vi "FT_Get_Device_Info.vi"(0 "Handle":u32) -> (1 "FT_Status":u32(ring) items=["FT_OK", "FT_INVALID_HANDLE", "FT_DEVICE_NOT_FOUND", "FT_DEVICE_NOT_OPENED", "FT_IO_ERROR", "FT_INSUFFICIENT_RESOURCES", "FT_INVALID_PARAMETER", "FT_INVALID_BAUD_RATE", "FT_DEVICE_NOT_OPENED_FOR_ERASE", "FT_DEVICE_NOT_OPENED_FOR_WRITE", "FT_FAILED_TO_WRITE_DEVICE", "FT_EEPROM_READ_FAILED", "FT_EEPROM_WRITE_FAILED", "FT_EEPROM_ERASE_FAILED", "FT_EEPROM_NOT_PRESENT", "FT_EEPROM_NOT_PROGRAMMED", "FT_INVALID_ARGS", "FT_NOT_SUPPORTED", "FT_OTHER_ERROR"], 2 "Device Information":T1 {"Type" items=["FT232B-FT245B", "FT8U232AM-FT8U245AM", "FT8U100AX", "UNKNOWN", "FT2232", "FT232R-FT245R", "FT2232H", "FT4232H", "FT232H"]})   [LabVIEW 2019, in "D2XX_Functions.lvlib"]
uses:
  <userlib>/LevyLab/Relay Box/D2XX_Functions/D2XX_Functions.lvlib
  <userlib>/LevyLab/Relay Box/D2XX_Functions/i386/ftd2xx.dll
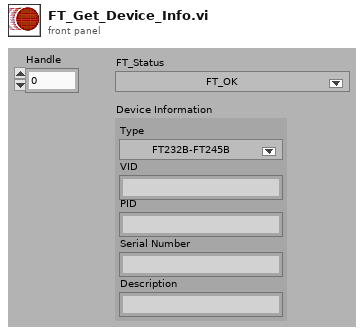
[diagram p1: front panel]
types:
  T1 = cluster{"Type":u32, "VID":string, "PID":string, "Serial Number":string, "Description":string}
  T2 = cluster{"DeviceType":u32, string, string, "SerialNumber":string, "Description":string}
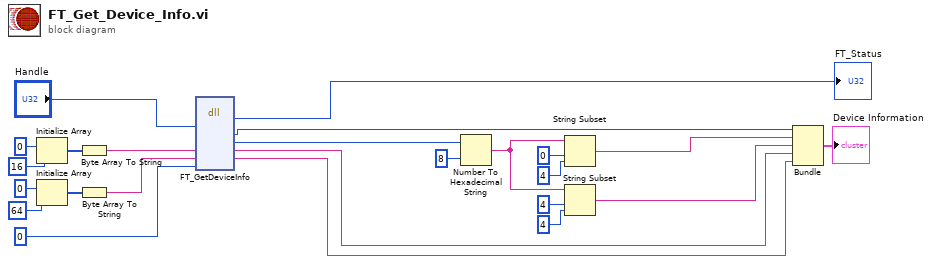
[diagram p0: block diagram]
diagram:
  n1 = Initialize Array(u8 0, 16 ("dimension size")) -> (w8:u8[])
  n2 = Initialize Array(u8 0, 64 ("dimension size")) -> (w6:u8[])
  n3 = Byte Array To String(unsigned byte array=w8) -> (string=w2:string)
  n4 = Byte Array To String(unsigned byte array=w6) -> (string=w3:string)
  n5 = dll-call lib="C:/Program Files (x86)/National Instruments/LabVIEW 2019/user.lib/LevyLab/Relay Box/D2XX_Functions/i386/FTD2XX.dll" fn="FT_GetDeviceInfo"("Handle"="Handle", "SerialNumber"=w2, "Description"=w3, "Dummy"=u32 0) -> ("FT_Status"=→"FT_Status":u32, "DeviceType"=w1:u32, "ID"=w22:u32, "SerialNumber"=w13:string, "Description"=w12:string)  [unwired: 7 in, 2 out]
  n6 = Number To Hexadecimal String(1:i16 8 ("width (-)"), 2:w22) -> (0:w16:string)
  n7 = String Subset(string=w16, offset (0)=0, length (rest)=4 ("length (rest)")) -> (substring=w15:string)
  n8 = String Subset(string=w16, offset (0)=4, length (rest)=4 ("length (rest)")) -> (substring=w14:string)
  n9 = Bundle("DeviceType"=w1, w15, w14, "SerialNumber"=w13, "Description"=w12) -> (→"Device Information":T2)  [unwired: 1 in]
